vi "host.vi"() -> ()   [LabVIEW 2010]
uses:
  <vilib>/userDefined/High Color/nirio_resource_hc.ctl
  <vilib>/rvi/interface/nirviOpenFPGA/nirviOpenFPGA.xnode
  FPGA Bitfiles/flexRIOTest_main.lvbitx
  <vilib>/rvi/ClientSDK/nirviWhatTheDeviceIsDoing.ctl
  <vilib>/rvi/interface/nirviMethod/nirviMethod.xnode
  <vilib>/rvi/interface/common/niFpgaNodeNameForErrorReporting.ctl
  <vilib>/rvi/errors/niLvFpgaWhatHappensToTopLevelVI.ctl
  <vilib>/rvi/interface/nirviCloseFPGA/nirviCloseFPGA.xnode
  <vilib>/FPGAPlugInAG/PXIe-7962R/niLvFpga_Open_PXIe-7962R.vi
  <vilib>/rvi/interface/common/dynamic/niFpgaDynamicAddResources.vi
  <vilib>/Utility/error.llb/Error Cluster From Error Code.vi
  <vilib>/rvi/errors/niLvFpgaAdjustHostInterfaceError.vi
  <vilib>/FPGAPlugInAG/Dynamic/niLvFpga_Close_Dynamic.vi
  NiFpgaLv.dll
panel:
  in  "stop":bool
  in  "Timeout (ms)":i32=1000
  out "Data":u16[](array[numeric])
  out "Elements Remaining":u32
  in  "Number of Elements":u32=20000
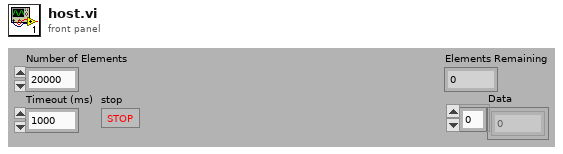
[diagram p1: front panel]
types:
  T1 = typedef "nirio_resource_hc.ctl" = tag
  T2 = typedef "niFpgaNodeNameForErrorReporting.ctl" = enum16{"Open FPGA VI Reference", "Read/Write Control", "Invoke Method: Abort", "Invoke Method: Acknowledge IRQ", "Invoke Method: Download", "Invoke Method: FIFO.Configure", "Invoke Method: FIFO.Read", "Invoke Method: FIFO.Start", "Invoke Method: FIFO.Stop", "Invoke Method: FIFO.Write", "Invoke Method: Reset", "Invoke Method: Run", "Invoke Method: Wait on IRQ", "Close FPGA VI Reference"}
  T3 = typedef "niLvFpgaWhatHappensToTopLevelVI.ctl" = enum16{"top level VI scripted behind XNode", "top level VI inlined behind XNode"}
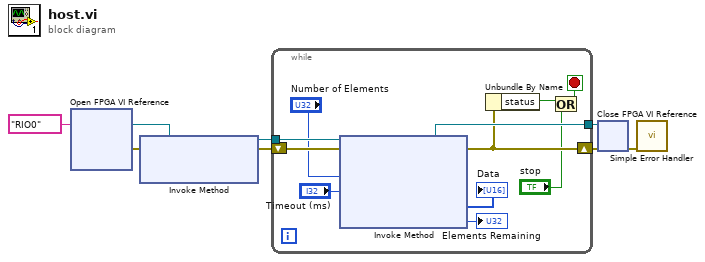
[diagram p0: block diagram]
diagram:
  n1 = xnode "Open FPGA VI Reference"("resource name"=T1 "RIO0") -> ("FPGA VI Reference Out"=w5:refnum<k20>, "error out"=w8:errorcluster)  [unwired: 1 in]
  n2 = xnode "Invoke Method"("FPGA VI Reference In"=w5, "error in"=w8) -> ("FPGA VI Reference Out"=w4:refnum<k20>, "error out"=w7:errorcluster)  [unwired: 1 in]
  n3 = while {
    shift-right: [w12] -> w6
    shift-left: w7 -> [w19]
    tunnel: w4 -> [w18]
    tunnel: [w17] -> w3
    stop <- w9 stop-if-true
    n4 = xnode "Invoke Method"("FPGA VI Reference In"=w18, "error in"=w19, "Number of Elements"="Number of Elements", "Timeout (ms)"="Timeout (ms)") -> ("FPGA VI Reference Out"=w17:refnum<k20>, "error out"=w12:errorcluster, "Data"=→"Data":u16[], "Elements Remaining"=→"Elements Remaining":u32)
    n5 = Unbundle By Name(w12) -> ("status"=w11:bool)
    n6 = Or(x=w11, y="stop") -> (x .or. y?=w9:bool)
  }
  n7 = xnode "Close FPGA VI Reference"("FPGA VI Reference In"=w3, "error in"=w6) -> ("error out"=w1:errorcluster)
  n8 = call <vilib>:"Simple Error Handler.vi"("error in (no error)"=w1) -> ()  [unwired: 4 in, 5 out]
